vi "APS absolute linear move.vi"(7 "Max_Linear_Speed":i32, 8 "error in (no error)":errorcluster caption="错误输入（无错误）", 9 "Position_Array":i32[](array[numeric]), 10 "Axis_ID_Array":i32[](array[numeric]), 11 "Dimension":i32) -> (0 "error out":errorcluster caption="错误输出", 1 "Position_Array 2":i32[](array[numeric]), 2 "Axis_ID_Array 2":i32[](array[numeric]), 3 "function return":i32)   [LabVIEW 2017, in "APS168.lvlib"]
doc: "I32 FNTYPE APS_absolute_linear_move( I32 Dimension, I32 *Axis_ID_Array, I32 *Position_Array, I32 Max_Linear_Speed );"
uses:
  APS168.lvlib
  APS168.dll
  Global/global-cj.vi
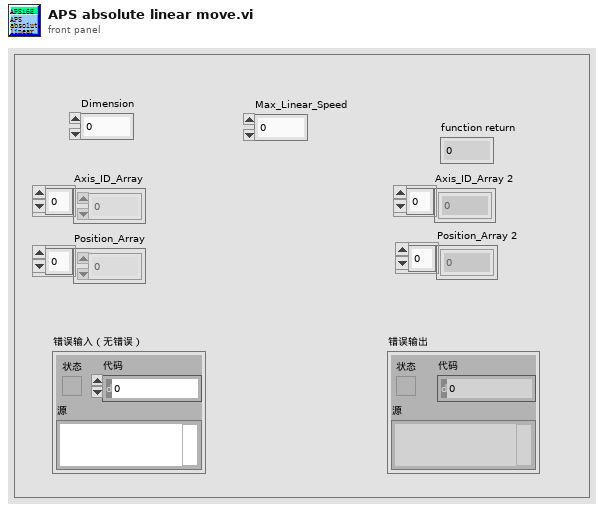
[diagram p1: front panel]
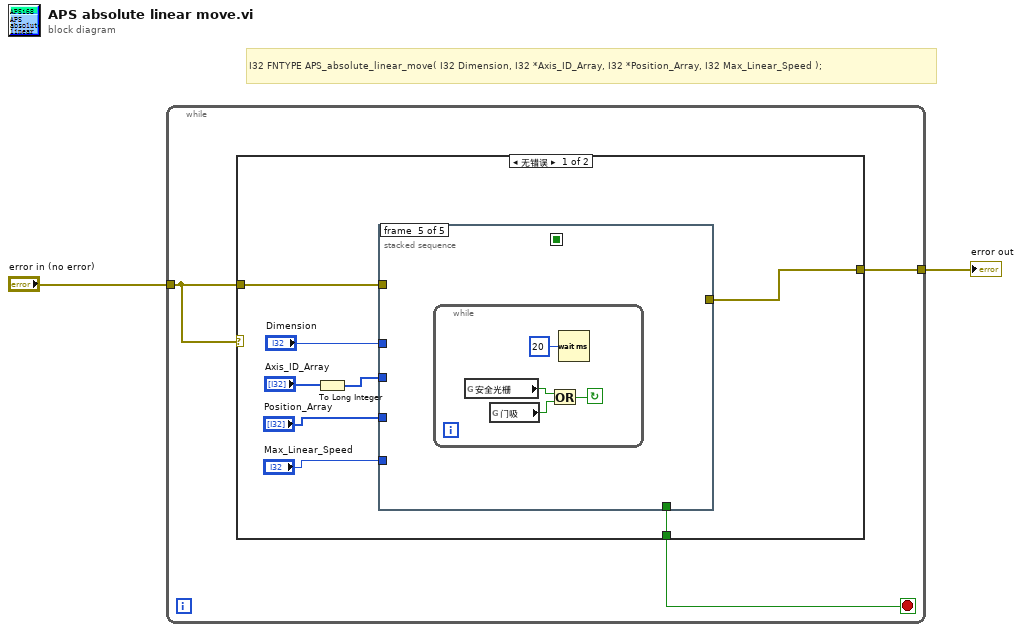
[diagram p0: block diagram]
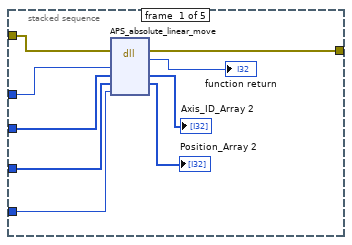
[diagram p2: hidden frame]
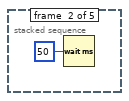
[diagram p3: hidden frame]
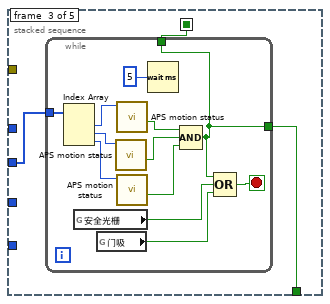
[diagram p4: hidden frame]
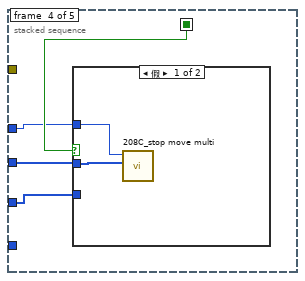
[diagram p5: hidden frame]
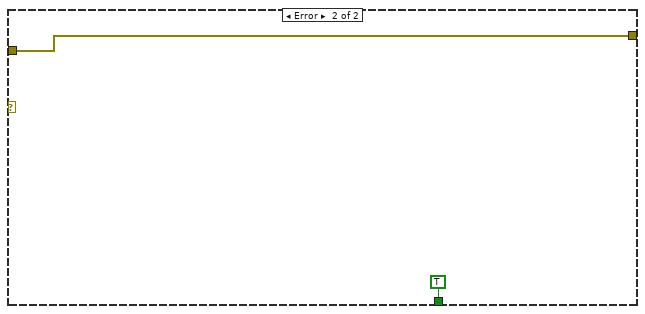
[diagram p7: hidden frame]
diagram:
  # "I32 FNTYPE APS_absolute_linear_move( I32 Dimension, I32 *Axis_ID_Array, I32 *Position_Array, I32 Max_Linear_Speed );"
  n1 = while {
    tunnel: [w5] -> w2
    tunnel: "error in (no error)" -> [w4]
    stop <- w3 stop-if-true
    n2 = case shown="无错误" w4 {
      tunnel: w4 -> [w13 w50]
      tunnel: [w12 w50] -> w5
      tunnel: [w7 TRUE] -> w3
      frame No Error {
        n3 = To Long Integer(number="Axis_ID_Array") -> (32bit integer=w6:i32[])
        n4 = stacked-sequence {
          seq-local: [_ _ w25 _ _] -> [_ _ _ w42 _]
          tunnel: "Position_Array" -> [w14 _ _ w41 _]
          tunnel: [_ _ w26 _ _] -> w7
          tunnel: w13 -> [w19 _ _ _ _]
          tunnel: [w18 _ _ _ _] -> w12
          tunnel: "Dimension" -> [w17 _ _ w40 _]
          tunnel: w6 -> [w16 _ w24 w39 _]
          tunnel: "Max_Linear_Speed" -> [w15 _ _ _ _]
          frame #0 {
            n5 = dll-call lib="PTH2Gabs E迈治LV范例testSubVIsADLINKMotion204cAPS168.*" fn="APS_absolute_linear_move"(error in=w19, "Dimension"=w17, "Axis_ID_Array"=w16, "Position_Array"=w14, "Max_Linear_Speed"=w15) -> (error out=w18:errorcluster, "return type"=→"function return":i32, "Axis_ID_Array"=→"Axis_ID_Array 2":i32[], "Position_Array"=→"Position_Array 2":i32[])  [unwired: 4 in, 1 out]
          }
          frame #1 {
            n6 = Wait (ms)(milliseconds to wait=u32 50 ("等待时间（毫秒）")) -> ()  [unwired: 1 out]
          }
          frame #2 {
            n7 = while {
              tunnel: w24 -> [w37]
              tunnel: [w30] -> w26
              tunnel: [w30] -> w25
              stop <- w27 stop-if-true
              n8 = Index Array(array=w37) -> (element #1=w36:i32, element #2=w35:i32, element #3=w34:i32)  [unwired: 3 in]
              n9 = global read "global-cj.vi" "安全光栅"() -> (w29:bool)
              n10 = global read "global-cj.vi" "门吸"() -> (w28:bool)
              n11 = call "APS motion status.vi"("Axis_ID"=w35) -> ("x与y?"=w32:bool)  [unwired: 9 in, 1 out]
              n12 = call "APS motion status.vi"("Axis_ID"=w36) -> ("x与y?"=w33:bool)  [unwired: 9 in, 1 out]
              n13 = call "APS motion status.vi"("Axis_ID"=w34) -> ("x与y?"=w31:bool)  [unwired: 9 in, 1 out]
              n14 = Wait (ms)(milliseconds to wait=u32 5 ("等待时间（毫秒）")) -> ()  [unwired: 1 out]
              n15 = Compound Arithmetic op=AND(w33, w32, w31) -> (w30:bool)
              n16 = Compound Arithmetic op=OR(w30, w29, w28) -> (w27:bool)
            }
          }
          frame #3 {
            n17 = case shown="假" w42 {
              tunnel: w41 -> [_ _]
              tunnel: w40 -> [w44 _]
              tunnel: w39 -> [w43 _]
              frame False {
                n18 = call "208C_stop move multi.vi"("Axis_ID_Array"=w43, "Dimension"=w44) -> ()  [unwired: 7 in, 3 out]
              }
              frame True {
              }
            }
          }
          frame #4 {
            n19 = while {
              stop <- w45 continue-if-true
              n20 = global read "global-cj.vi" "安全光栅"() -> (w47:bool)
              n21 = global read "global-cj.vi" "门吸"() -> (w46:bool)
              n22 = Or(x=w47, y=w46) -> (x .or. y?=w45:bool)
              n23 = Wait (ms)(milliseconds to wait=u32 20 ("等待时间（毫秒）")) -> ()  [unwired: 1 out]
            }
          }
        }
      }
      frame Error {
      }
    }
  }
  "error out" <- w2
